vi "Read Multi-Channel Waveform.vi"(8 "error in (no error)":errorcluster, 10 "Channels":T1[](array[typedef]), 11 "MSOX6004 in":refnum<class "MSOX6004.lvclass">) -> (0 "error out":errorcluster, 2 "Waveform":waveform(dbl)[](graph), 3 "MSOX6004 out":refnum<class "MSOX6004.lvclass">)   [LabVIEW 2018, in "MSOX6004.lvlib" / "MSOX6004.lvclass"]
doc: "This Override method is used to initiate multi-channel waveform acquisition. Select targeted channels at the 'Channels' control and output waveform data to the 'Waveform' indicator."
uses:
  MSOX6004.lvclass
  PPLs/Oscilloscope/Parent/Oscilloscope.lvlibp/Custom Controls/Analog Channels.ctl
  PPLs/Oscilloscope/Parent/Oscilloscope.lvlibp
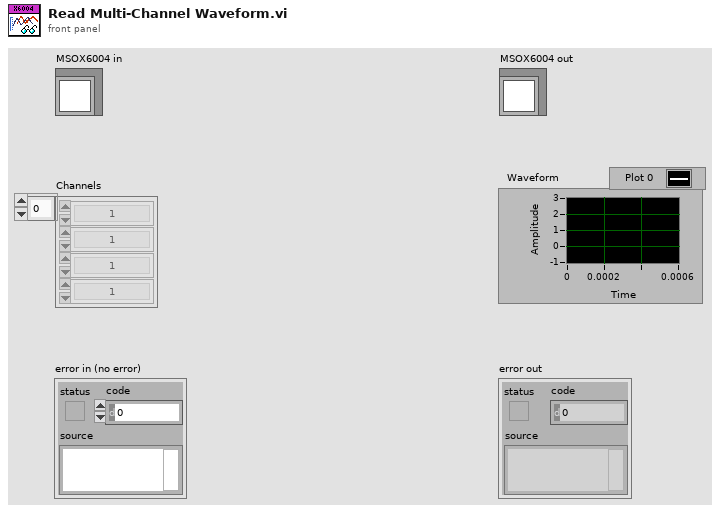
[diagram p1: front panel]
types:
  T1 = typedef "Oscilloscope.lvlibp/Analog Channels.ctl" = enum16{"1", "2", "3", "4", "5", "6", "7", "8", "9", "10", "11", "12", "13", "14", "15", "16"}
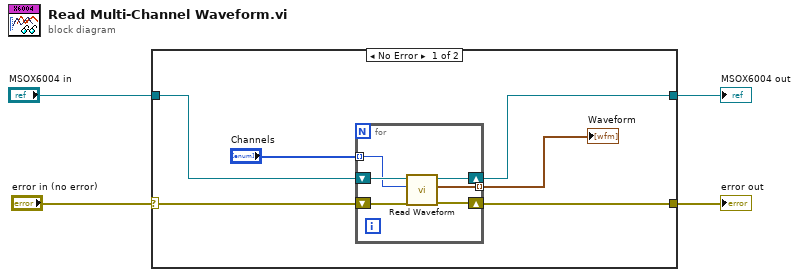
[diagram p0: block diagram]
diagram:
  n1 = case shown="No Error" "error in (no error)" {
    selector: "error in (no error)" -> [w6 w18]
    tunnel: [w8 w18] -> w3
    tunnel: [w9 w17] -> w2
    tunnel: "MSOX6004 in" -> [w5 w17]
    frame No Error {
      n2 = for {
        tunnel: "Channels" -> [w14] mode=indexing
        shift-right: [w13] -> w9
        shift-left: w5 -> [w16]
        shift-right: [w12] -> w8
        shift-left: w6 -> [w15]
        tunnel: [w11] -> w7 mode=indexing
        n3 = call-dynamic "Read Waveform.vi"("error in (no error)"=w15, "Channel"=w14, "MSOX6004 in"=w16) -> ("error out"=w12:errorcluster, "Waveform"=w11:waveform(dbl), "MSOX6004 out"=w13:refnum<class "MSOX6004.lvclass">)  [unwired: 6 in]
      }
      "Waveform" <- w7
    }
    frame Error {
    }
  }
  "error out" <- w3
  "MSOX6004 out" <- w2
